vi "TankSelectCtl.vi"(6 "pump":bool, 8 "enable":bool, 9 "valve t-2 close":bool, 10 "valve t-1 close":bool, 11 "Tank":bool) -> (2 "valve t-2":bool, 3 "valve t-1":bool)   [LabVIEW 2011]
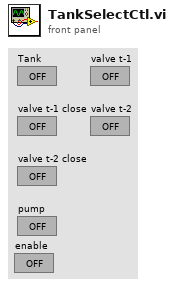
[diagram p1: front panel]
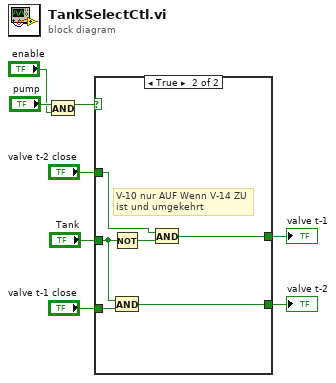
[diagram p0: block diagram]
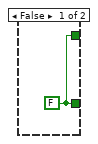
[diagram p2: hidden frame]
diagram:
  n1 = And(x="pump", y="enable") -> (x .and. y?=w2:bool)
  n2 = case shown="True" w2 {
    tunnel: "Tank" -> [_ w13]
    tunnel: "valve t-2 close" -> [_ w15]
    tunnel: "valve t-1 close" -> [_ w12]
    tunnel: [w9 w11] -> w7
    tunnel: [w9 w10] -> w8
    frame False {
      w9 = FALSE
    }
    frame True {
      # "V-10 nur AUF Wenn V-14 ZU\nist und umgekehrt"
      n3 = Not(x=w13) -> (.not. x?=w14:bool)
      n4 = And(x=w13, y=w12) -> (x .and. y?=w10:bool)
      n5 = And(x=w15, y=w14) -> (x .and. y?=w11:bool)
    }
  }
  "valve t-2" <- w8
  "valve t-1" <- w7
